vi "FileUpdater.vi"   [LabVIEW 2014]
uses:
  Robot Global Data.vi
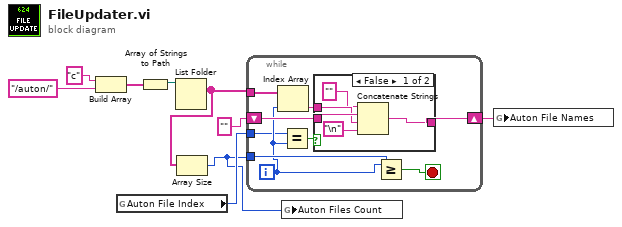
[diagram p0: block diagram]
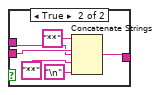
[diagram p2: hidden frame]
diagram:
  n1 = Build Array("c", "/auton/") -> (w5:string[])
  n2 = global read "Robot Global Data.vi" "Auton File Index"() -> (w2:i32)
  n3 = Array of Strings to Path(0:w5) -> (2:w6:path)  [unwired: 1 in]
  n4 = List Folder(path=w6) -> (filenames=w4:string[])  [unwired: 3 in, 3 out]
  n5 = Array Size(array=w4) -> (size(s)=w1:i32)
  n6 = while {
    tunnel: w4 -> [w16]
    tunnel: w1 -> [w17]
    shift-right: [w15] -> w3
    shift-left: "" -> [w14]
    tunnel: w2 -> [w10]
    i -> [w11]
    stop <- w18 stop-if-true
    n7 = Index Array(array=w16, index=w11) -> (element=w13:string)
    n8 = Equal?(x=w10, y=w11) -> (x = y?=w12:bool)
    n9 = case shown="False" w12 {
      tunnel: [w23 w26] -> w15
      tunnel: w14 -> [w22 w29]
      tunnel: w13 -> [w21 w28]
      frame False {
        n10 = Concatenate Strings("" ("string"), w22, w21, "\n") -> (w23:string)
      }
      frame True {
        n11 = Concatenate Strings("**" ("string"), w29, w28, "**" ("string"), "\n") -> (w26:string)
      }
    }
    n12 = Greater Or Equal?(x=w11, y=w17) -> (x >= y?=w18:bool)
  }
  n13 = global write "Robot Global Data.vi" "Auton Files Count"(w1) -> ()
  n14 = global write "Robot Global Data.vi" "Auton File Names"(w3) -> ()
